vi "GenerateLibraryBanner.vi"(8 "error in (no error)":errorcluster, 9 "Text settings":T1={"Size"=8, "Capitalize text"=TRUE, "TextColor"=0}, 10 "Rectangle colors (black, white)":T2={"Border"=0, "Background"=4643840}, 11 "Text":string) -> (0 "error out":errorcluster, 2 "Picture":picture, 3 "Icon.lvlclass out":refnum<class "Icon.lvclass">)   [LabVIEW 2014, in "ClassIconTools.lvlib"]
doc: "Basic example that shows how to set the Template Layer."
uses:
  ClassIconTools.lvlib
  <vilib>/LabVIEW Icon API/lv_icon/Classes/Icon/Icon.lvclass
  <vilib>/LabVIEW Icon API/API_Rectangle Colors.ctl
  <vilib>/LabVIEW Icon API/API_Rectangle Dimension.ctl
  <vilib>/LabVIEW Icon API/API_Text.ctl
  <vilib>/LabVIEW Icon API/API_Test Settings.ctl
  <vilib>/LabVIEW Icon API/lv_icon/Controls/Alignment.ctl
  <vilib>/LabVIEW Icon API/API_Text Colors.ctl
  <vilib>/LabVIEW Icon API/LabVIEW Icon API.lvlib
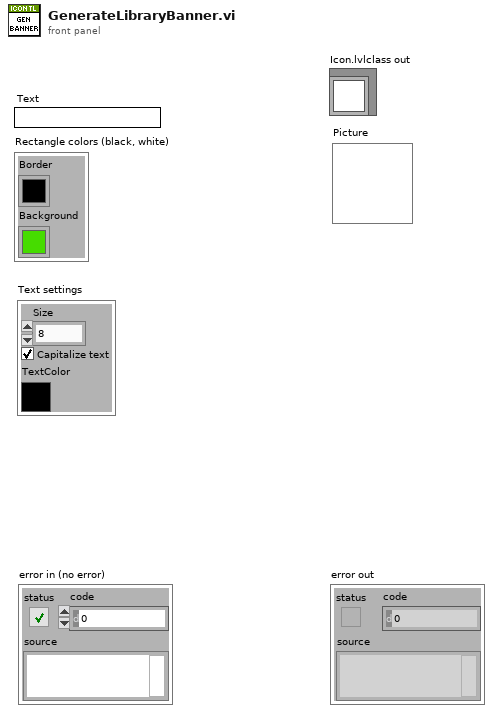
[diagram p1: front panel]
types:
  T1 = cluster{"Size":u8, "Capitalize text":bool, "TextColor":u32}
  T2 = typedef "LabVIEW Icon API.lvlib/API_Rectangle Colors.ctl" = cluster{"Border":u32, "Background":u32}
  T3 = typedef "LabVIEW Icon API.lvlib/API_Test Settings.ctl" = cluster{"Font":string, "Alignment":T4, "Size":u8, "Center text":bool, "Capitalize text":bool, "Text color":T5}
  T4 = typedef "Alignment.ctl" = u16
  T5 = typedef "LabVIEW Icon API.lvlib/API_Text Colors.ctl" = cluster{"Line 1 color":u32, "Line 2 color":u32, "Line 3 color":u32, "Line 4 color":u32}
  T6 = typedef "LabVIEW Icon API.lvlib/API_Text.ctl" = cluster{"Line 1 text":string, "Line 2 text":string, "Line 3 text":string, "Line 4 text":string}
  T7 = typedef "LabVIEW Icon API.lvlib/API_Rectangle Dimension.ctl" = cluster{"Width":i16, "Height":i16}
  T8 = typedef "imagedata.ctl" = cluster{"image type":i32, "image depth":i32, "image":u8[], "mask":u8[], "colors":u32[], "Rectangle":cluster{"left":i16, "top":i16, "right":i16, "bottom":i16}}
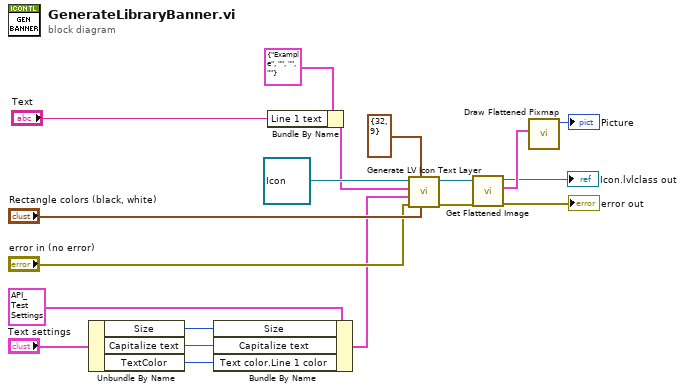
[diagram p0: block diagram]
diagram:
  n1 = Unbundle By Name("Text settings") -> ("Size"=w3:u8, "Capitalize text"=w2:bool, "TextColor"=w1:u32)
  n2 = Bundle By Name(cluster=T3 {"Font"="Small Fonts", "Alignment"=1, "Size"=8, "Center text"=TRUE, "Capitalize text"=TRUE, "Text color"={"Line 1 color"=0, "Line 2 color"=0, "Line 3 color"=0, "Line 4 color"=0}} ("Text settings"), "Size"=w3, "Capitalize text"=w2, "Text color.Line 1 color"=w1) -> (w5:T3)
  n3 = Bundle By Name(cluster=T6 {"Line 1 text"="Example", "Line 2 text"="", "Line 3 text"="", "Line 4 text"=""} ("Text"), "Line 1 text"="Text") -> (w9:T6)
  n4 = call <vilib>:"Generate LV Icon Text Layer.vi"("Rectangle colors (black, white)"="Rectangle colors (black, white)", "Rectangle dimension (32,32)"=T7 {"Width"=32, "Height"=9}, "error in (no error)"="error in (no error)", "Text settings"=w5, "Text"=w9, "Icon in"=refnum<class "Icon.lvclass"> refnum ("Icon.lvclass in")) -> ("error out"=w10:errorcluster, "Icon out"=w11:refnum<class "Icon.lvclass">)  [unwired: 4 in]
  n5 = call <vilib>:"Get Flattened Image.vi"("error in (no error)"=w10, "lv_icon.lvlib:Icon.lvclass in"=w11) -> ("error out"=→"error out":errorcluster, "Color Image"=w19:T8, "lv_icon.lvlib:Icon.lvclass out"=→"Icon.lvlclass out":refnum<class "Icon.lvclass">)  [unwired: 6 in, 1 out]
  n6 = call <vilib>:"Draw Flattened Pixmap.vi"("image data"=w19) -> ("new picture"=→"Picture":picture)  [unwired: 8 in]
